vi "Draw Interface.vi"(8 "Interface elevation":dbl, 9 "Interface inputs":T2={"Elevation of top of Field of View (cm)"=10.0, "Field of View Height (cm)"=-0.1, "Smooth Length (cm)"=5.0, "Min derivative magnitude"=5.0, "Color Plane"=enum."Green"} {"Smooth Length (cm)" min=0.01 max=1000.0 step=0.1; "Field of View Height (cm)" min=0.1 max=1000.0 step=0.1}, 10 "Image Dst":T1, 11 "Image":T1(plugin-control)=refnum) -> (3 "Image out":T1(plugin-control))   [LabVIEW 2012]
uses:
  Process Controller 3.0/Control code/Camera/Camera source code/Interface Inputs.ctl
  <vilib>/vision/Image Controls.llb/IMAQ Image.ctl
  <vilib>/vision/NI_Vision_Development_Module.lvlib
  <resource>/objmgr/IMAQImage.rc
  Process Controller 3.0/Control code/Camera/Camera SubVIs.lvlib
panel:
  out "Coordinates":i32[](array[numeric])
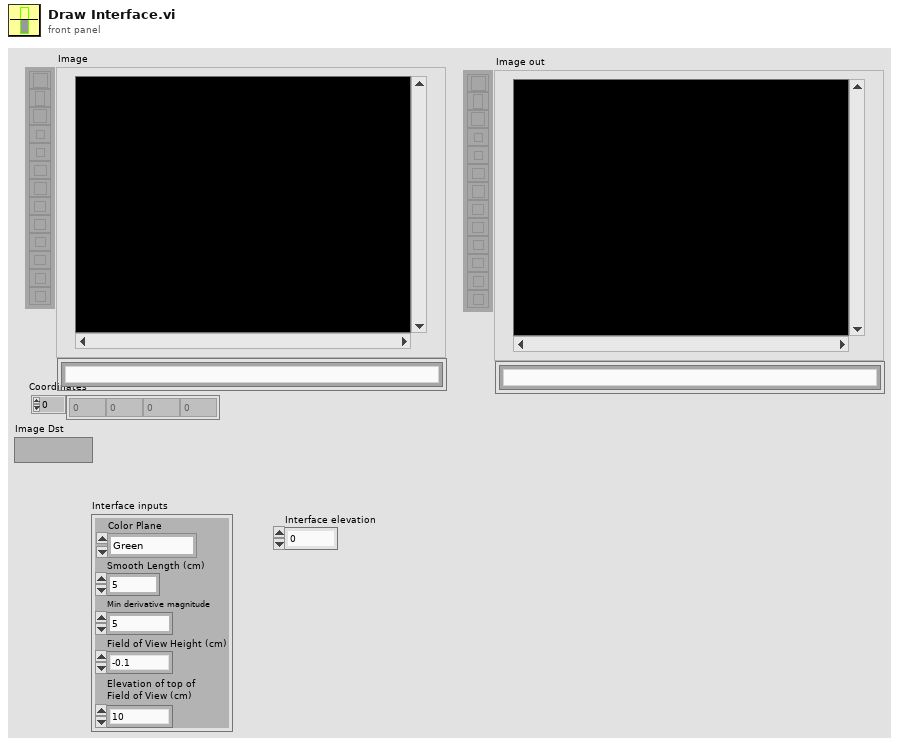
[diagram p1: front panel]
types:
  T1 = typedef "IMAQ Image.ctl" = refnum<image>
  T2 = typedef "Camera SubVIs.lvlib/Interface Inputs.ctl" = cluster{"Elevation of top of Field of View (cm)":dbl, "Field of View Height (cm)":dbl, "Smooth Length (cm)":dbl, "Min derivative magnitude":dbl, "Color Plane":enum16{"Red", "Green", "Blue", "Combined"}}
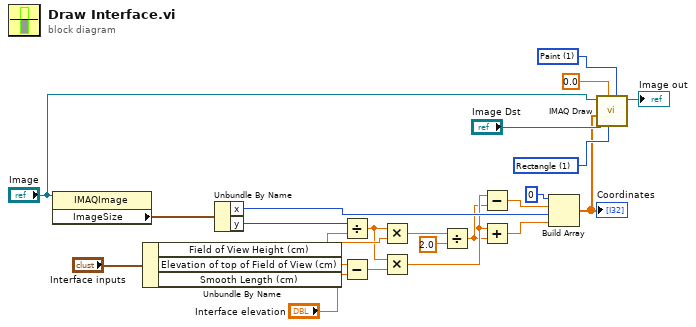
[diagram p0: block diagram]
diagram:
  w21 = u16 1 items=["Frame", "Paint", "Invert Frame", "Invert Paint"] ("Draw Mode")
  w23 = u16 1 items=["Line", "Rectangle", "Oval"] ("Shape to draw")
  n1 = property class="IMAQImage"(reference="Image") -> ("ImageSize"=w18:cluster{"x":i32, "y":i32})  [unwired: 1 in, 2 out]
  n2 = Unbundle By Name("Interface inputs") -> ("Field of View Height (cm)"=w13:dbl, "Elevation of top of Field of View (cm)"=w12:dbl, "Smooth Length (cm)"=w9:dbl)
  n3 = Unbundle By Name(w18) -> ("x"=w17:i32, "y"=w14:i32)
  n4 = Divide(x=w14, y=w13) -> (x/y=w8:dbl)
  n5 = Subtract(x=w12, y="Interface elevation") -> (x-y=w10:dbl)
  n6 = Multiply(x=w8, y=w9) -> (x*y=w7:dbl)
  n7 = Multiply(x=w8, y=w10) -> (x*y=w3:dbl)
  n8 = Divide(x=w7, y=2.0) -> (x/y=w2:dbl)
  n9 = Subtract(x=w3, y=w2) -> (x-y=w5:dbl)
  n10 = Add(x=w3, y=w2) -> (x+y=w1:dbl)
  n11 = Build Array(0 ("element"), w5, w17, w1) -> (w4:dbl[])
  "Coordinates" <- w4
  n12 = call "IMAQ Draw"("Draw Mode"=w21, "Shape to draw"=w23, "Pixel Color"=sgl 0.0, "Coordinates"=w4, "Image Dst"="Image Dst", "Image Src"="Image") -> ("Image Dst Out"=→"Image out":T1)  [unwired: 4 in, 1 out]
